vi "BlueSimpleReachTask 2.vi"() -> ()   [LabVIEW 2010]
uses:
  <vilib>/sound2/lvsound2.llb/Sound Data Format.ctl
  <vilib>/sound2/lvsound2.llb/Sampling Mode.ctl
  Controls/Bits to Write.ctl
  <vilib>/sound2/lvsound2.llb/Sound Output Set Volume (Single).vi
  <vilib>/sound2/lvsound2.llb/Sound Output Write (DBL Single).vi
  <vilib>/measure/NI_MABase.lvlib
panel:
  in  "Time to wait\nbefore treat \nArm freeze (S)":dbl=5.0
  in  "Arm Freeze \nCounter":bool
  in  "Volume":dbl(slide)=70.40816326530613 scale=0.0..100.0
  in  "Frequency":dbl=500.0 format="%0.2p"
  in  "error in (no error)":errorcluster
  in  "Sound Format":T1={"sample rate (S/s)"=44100.0, "number of channels"=2, "bits per sample"=16}
  in  "Number of Samples/ch":i32=5000
  in  "Device ID":u32
  in  "Catch Trial":bool
  in  "Catch probability":i32 min=0 max=100 step=1
  out "Catch Trial?":bool
  out "DO Task":refnum<k21>="BlueSimple_DO_All"
  out "DI Task":refnum<k21>="BlueSimple_DI"
  out "Exp correct":i32
  out "Record flag":bool
  in  "Recenter motor":bool
  in  "Override bumps":bool
  in  "Start bump timer?":bool
  in  "Trial type":u16(ring) items=["Allflash/sensory", "Precue/memory"]
  in  "DBS On?":bool
  in  "Home+target OK?":bool
  out "Exp reset":bool
  out "target set #":i32
  in  "duration (s)":dbl=0.18 format="%.4f"
  in  "Inter-pulse delay":cluster{"Fix":dbl, "Rnd":dbl}={"Fix"=0.0, "Rnd"=1.5} {"Rnd" format="%.4f"; "Fix" format="%_4g"}
  in  "Autofeed?":bool
  out "Just initialized\nhold loop?":bool
  in  "Home reward?":bool
  in  "Home  reward":cluster{"Fix":dbl, "Rnd":dbl} {"Rnd" format="%.4f"; "Fix" format="%_4g"}
  in  "Override 4":bool caption="Override 1"
  in  "Override 3":bool caption="Override 1"
  in  "Override 2":bool=TRUE caption="Override 1"
  in  "Override 1":bool=TRUE
  in  "LED lines":T2={"LED1"=1, "LED2"=2, "LED3"=3, "LED4"=4}
  in  "LED1":i16=5
  in  "LED2":i16=6
  in  "LED3":i16=7
  in  "LED4":i16=8
  in  "Bump Parameters":T3={"Distance (deg)"=2.0, "Travel time (ms)"=500.0} {"Travel time (ms)" min=0.1 max=10000.0; "Distance (deg)" min=0.1}
  in  "Bump delay":cluster{"Fix":dbl, "Rnd":dbl}={"Fix"=2.0, "Rnd"=8.0} {"Rnd" format="%.4f"; "Fix" format="%_4g"}
  in  "Sine parameters":T4={"Frequency"=1.0, "Degrees\npk-pk"=8.0, "Cycles"=10000} {"Degrees\npk-pk" min=0.1 max=120.0; "Frequency" min=0.001 format="%#_4g"}
  in  "Home":bool
  in  "Bumps":bool
  in  "Sines?":bool
  out "target set size":i32
  out "# target sets":u16
  in  "# Cycles":i16=20
  out "Instruct duration":dbl format="%.4f"
  out "Pre-I hold":dbl format="%.4f"
  out "Touching target\nlast time?":bool
  in  "Rand/Seq?":bool=TRUE
  in  "Target set":i16[](array[ring]) items=["1", "2", "3", "4"]
  in  "Block":T5(array[cluster])=array[6501 elements]
  in  "Settings In":T6={"Pre-I hold"={"Fixed (s)"=0.5, "Random (s)"=0.5}, "LED I duration"={"Fixed (s)"=0.5, "Random (s)"=0.0}, "All Flash?"=FALSE, "Pre-cue brightness"=0, "Post-I hold"={"Fixed (s)"=0.7, "Random (s)"=0.3}, "Post-I \nbounce-off"={"Fixed (s)"=0.3, "Random (s)"=0.0}, "Capture timeout"={"Fixed (s)"=1.5, "Random (s)"=0.0}, "Tone duration"={"Fixed (s)"=0.5, "Random (s)"=0.0}, "LED C duration"={"Fixed (s)"=0.5, "Random (s)"=0.0}, "Cue brightness"=0, "Hold duration"={"Fixed (s)"=0.3, "Random (s)"=0.0}, "Allowed\nbounce-off"={"Fixed (s)"=0.2, "Random (s)"=0.0}, "Post-capture brightness"=0, "Reward duration"={"Fixed (s)"=0.7, "Random (s)"=0.0}, "Intertrial interval"={"Fixed (s)"=0.5, "Random (s)"=0.0}, "Persistent Mode?"=FALSE, "Error bong?"=TRUE, "Critter"=0, "Blocks"=[], "Target set"=[], "Rand/Seq?"=TRUE, "Trial type"=0, "Sines?"=FALSE, "Bumps"=FALSE, "Sine parameters"={"Frequency"=0.25, "Degrees\npk-pk"=6.0, "Cycles"=10000}, "Bump timing"={"Fix"=2.0, "Rnd"=8.0}, "Bump Parameters"={"Distance (deg)"=2.0, "Travel time (ms)"=500.0}, "DBS On?"=FALSE, "Home reward?"=FALSE, "Home+target OK?"=FALSE} {"Bump Parameters"."Travel time (ms)" min=0.1 max=10000.0; "Bump Parameters"."Distance (deg)" min=0.1; "Bump timing"."Rnd" format="%.4f"; "Bump timing"."Fix" format="%_4g"; "Sine parameters"."Degrees\npk-pk" min=0.1 max=120.0; "Sine parameters"."Frequency" min=0.001 format="%#_4g"; "Trial type" items=["Allflash/sensory", "Precue/memory"]; "Target set" items=["1", "2", "3", "4"]; "Critter" items=["Mojo", "Smokey"]; "Post-I \nbounce-off"."Random (s)" format="%.4f"; "Post-I \nbounce-off"."Fixed (s)" format="%_4g"; "Allowed\nbounce-off"."Random (s)" format="%.4f"; "Allowed\nbounce-off"."Fixed (s)" format="%_4g"; "LED C duration"."Random (s)" format="%.4f"; "LED C duration"."Fixed (s)" format="%.4f"; "Capture timeout"."Random (s)" format="%.4f"; "Capture timeout"."Fixed (s)" format="%.4f"; "Post-I hold"."Random (s)" format="%.4f"; "Post-I hold"."Fixed (s)" format="%.4f"; "Hold duration"."Random (s)" format="%.4f"; "Hold duration"."Fixed (s)" format="%_4g"; "Intertrial interval"."Random (s)" format="%.4f"; "Intertrial interval"."Fixed (s)" format="%.4f"; "Reward duration"."Random (s)" format="%.4f"; "Reward duration"."Fixed (s)" format="%.4f"; "LED I duration"."Random (s)" format="%.4f"; "LED I duration"."Fixed (s)" format="%.4f"; "Tone duration"."Random (s)" format="%.4f"; "Tone duration"."Fixed (s)" format="%.4f"; "Pre-I hold"."Random (s)" format="%.4f"; "Pre-I hold"."Fixed (s)" format="%_4g"}
  in  "pause":bool
  out "Assign settings":bool
  out "current path":path
  out "next trial path":path
  in  "Critter":u16(ring) items=["Mojo", "Smokey", "Blue", "Odo", "Monk 5", "Monk 6", "Monk 7", "Monk 8", "Monk 9", "Monk 10"]
  out "Total incorrect":i32
  in  "Write Settings":bool
  in  "Read Settings":bool
  in  "All Flash?":bool
  in  "Post-capture brightness":i16 caption="Brightness"
  in  "Cue brightness":i16=6 caption="Brightness"
  in  "Pre-cue brightness":i16 caption="Brightness"
  out "Total correct":i32
  out "Total %":dbl
  out "Total trials":i32
  in  "Error\nbong?":bool=TRUE
  out "TS Home":bool
  out "TS 4":bool
  out "TS 3":bool
  out "TS 2":bool
  out "TS 1":bool
  out "Waveform Chart":T7(graph)
  out "Block trials":i32
  out "Block %":dbl
  in  "Reset\ncounters":bool
  in  "Post-I \nbounce-off":cluster{"Fix":dbl, "Rnd":dbl}={"Fix"=0.3, "Rnd"=0.0} caption="Allowed\nbounce-off" {"Rnd" format="%.4f"; "Fix" format="%_4g"}
  out "Exp trials":i32
  out "Exp %":dbl
  in  "Touch lines":T8={"Home touch"=0, "Touch 1"=1, "Touch 2"=2, "Touch 3"=3, "Touch 4"=4}
  out "Current stage":T9(ring)
  in  "Allowed\nbounce-off":cluster{"Fix":dbl, "Rnd":dbl}={"Fix"=0.2, "Rnd"=0.0} {"Rnd" format="%.4f"; "Fix" format="%_4g"}
  in  "LED C duration":cluster{"Fix":dbl, "Rnd":dbl}={"Fix"=0.5, "Rnd"=0.0} caption="LED duration" {"Rnd" format="%.4f"; "Fix" format="%.4f"}
  in  "Capture timeout":cluster{"Fix":dbl, "Rnd":dbl}={"Fix"=1.5, "Rnd"=0.0} caption="Response time" {"Rnd" format="%.4f"; "Fix" format="%.4f"}
  in  "Post-I hold":cluster{"Fix":dbl, "Rnd":dbl}={"Fix"=0.5, "Rnd"=0.5} {"Rnd" format="%.4f"; "Fix" format="%.4f"}
  out "Last trial successful?":bool
  in  "Persistent\n Mode?":bool
  in  "Touch 4":i16=4
  in  "Touch 3":i16=3
  in  "Touch 2":i16=2
  in  "Touch 1":i16=1
  in  "Home touch":i16
  in  "Hold duration":cluster{"Fix":dbl, "Rnd":dbl}={"Fix"=0.3, "Rnd"=0.0} {"Rnd" format="%.4f"; "Fix" format="%_4g"}
  out "Target":i16
  in  "stop":bool
  in  "device":i16=1
  in  "line direction map":i32=2147483616 format="%.0b"
  out "DIGIO task ID":u32 format="%.0x"
  out "error out":errorcluster
  in  "Intertrial interval":cluster{"Fix":dbl, "Rnd":dbl}={"Fix"=0.5, "Rnd"=0.0} {"Rnd" format="%.4f"; "Fix" format="%.4f"}
  in  "Reward duration":cluster{"Fix":dbl, "Rnd":dbl}={"Fix"=0.7, "Rnd"=0.0} {"Rnd" format="%.4f"; "Fix" format="%.4f"}
  in  "LED I duration":cluster{"Fix":dbl, "Rnd":dbl}={"Fix"=0.5, "Rnd"=0.0} caption="LED duration" {"Rnd" format="%.4f"; "Fix" format="%.4f"}
  in  "Tone duration":cluster{"Fix":dbl, "Rnd":dbl}={"Fix"=0.5, "Rnd"=0.0} {"Rnd" format="%.4f"; "Fix" format="%.4f"}
  in  "Pre-I hold":cluster{"Fix":dbl, "Rnd":dbl}={"Fix"=0.5, "Rnd"=0.5} {"Rnd" format="%.4f"; "Fix" format="%_4g"}
  # "Auto-feed"
  # "DBS"
  # "Pre-\ninstruction\nhold"
  # "Post-\ninstruction\nhold"
  # "Instruction"
  # "Target capture"
  # "Target hold"
  # "Reward"
  # "Intertrial"
  # "Motor"
  # "Override"
  # "Home key tone"
  # "+"
  # "+"
  # "+"
  # "Pre-\ninstruction\nhold"
  # "Instruction"
  # "Post-\ninstruction\nhold"
  # "Target capture"
  # "Target hold"
  # "Reward"
  # "Intertrial"
  # "+"
  # "+"
  # "+"
  # "+"
  # "+"
  # "+"
  # "+"
  # "+"
  # "+"
  # "+"
  # "+"
  # "+"
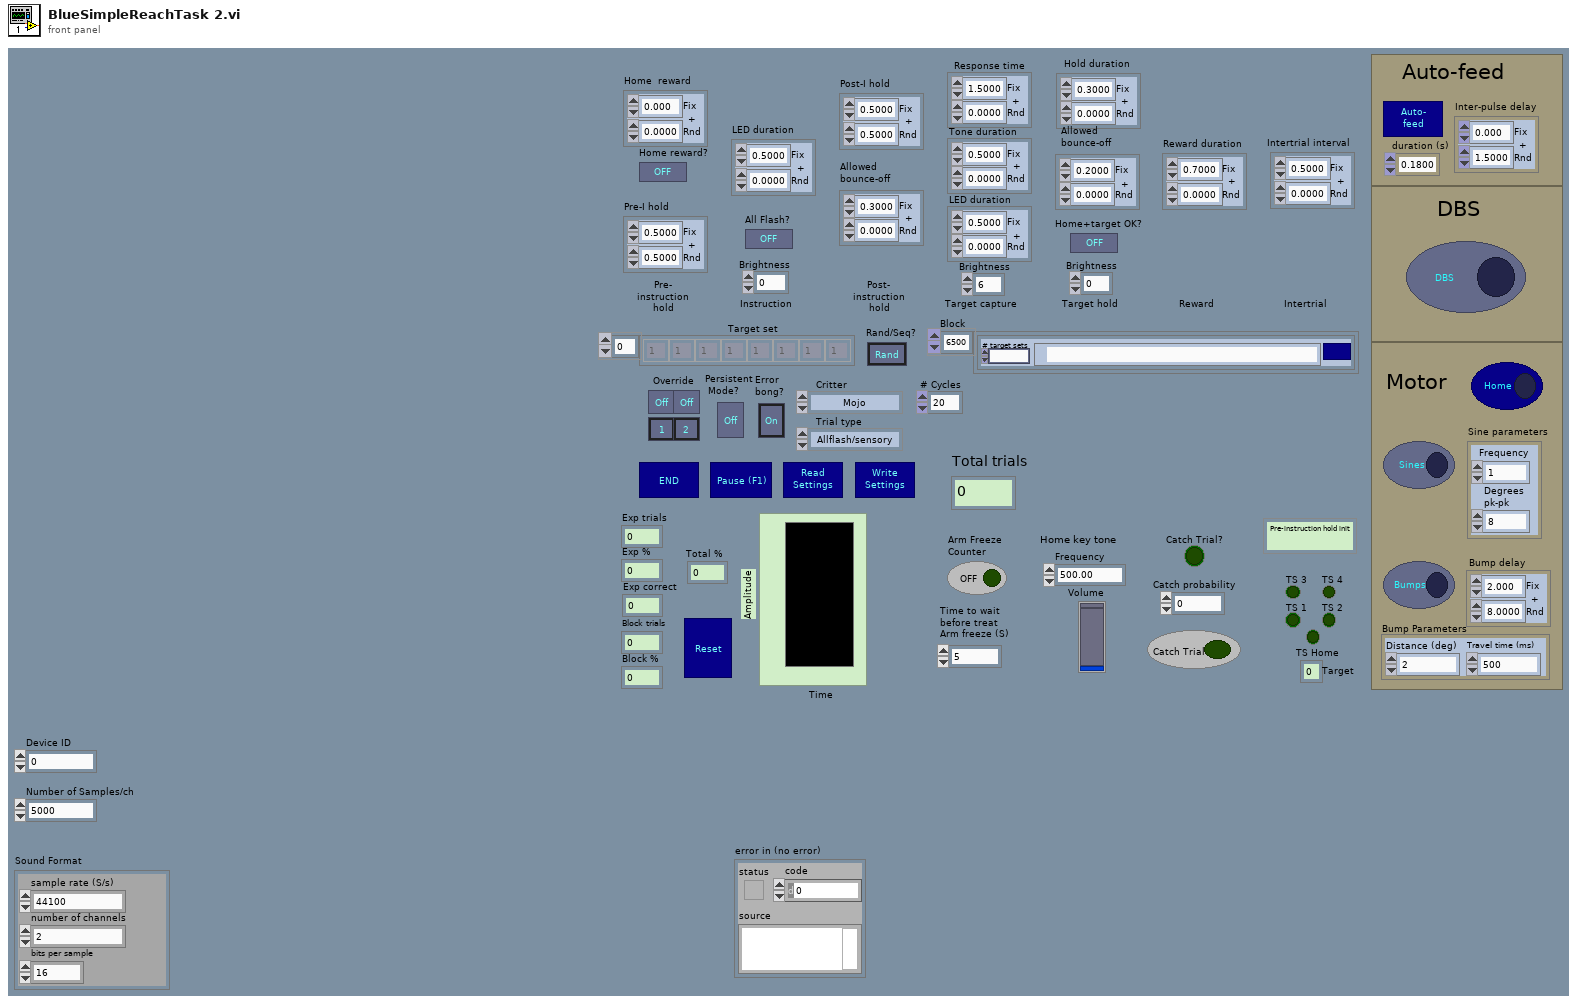
[diagram p1: front panel]
types:
  T1 = typedef "Sound Data Format.ctl" = cluster{"sample rate (S/s)":dbl, "number of channels":i32, "bits per sample":i32}
  T2 = cluster{"LED1":i16, "LED2":i16, "LED3":i16, "LED4":i16}
  T3 = cluster{"Distance (deg)":dbl, "Travel time (ms)":dbl}
  T4 = cluster{"Frequency":dbl, "Degrees\npk-pk":dbl, "Cycles":i16}
  T5 = cluster{"Settings file":path, "# target sets":u16}[]
  T6 = cluster{"Pre-I hold":cluster{"Fixed (s)":dbl, "Random (s)":dbl}, "LED I duration":cluster{"Fixed (s)":dbl, "Random (s)":dbl}, "All Flash?":bool, "Pre-cue brightness":i16, "Post-I hold":cluster{"Fixed (s)":dbl, "Random (s)":dbl}, "Post-I \nbounce-off":cluster{"Fixed (s)":dbl, "Random (s)":dbl}, "Capture timeout":cluster{"Fixed (s)":dbl, "Random (s)":dbl}, "Tone duration":cluster{"Fixed (s)":dbl, "Random (s)":dbl}, "LED C duration":cluster{"Fixed (s)":dbl, "Random (s)":dbl}, "Cue brightness":i16, "Hold duration":cluster{"Fixed (s)":dbl, "Random (s)":dbl}, "Allowed\nbounce-off":cluster{"Fixed (s)":dbl, "Random (s)":dbl}, "Post-capture brightness":i16, "Reward duration":cluster{"Fixed (s)":dbl, "Random (s)":dbl}, "Intertrial interval":cluster{"Fixed (s)":dbl, "Random (s)":dbl}, "Persistent Mode?":bool, "Error bong?":bool, "Critter":u16, "Blocks":cluster{"Settings file":path, "# target sets":dbl}[], "Target set":i16[], "Rand/Seq?":bool, "Trial type":u16, "Sines?":bool, "Bumps":bool, "Sine parameters":cluster{"Frequency":dbl, "Degrees\npk-pk":dbl, "Cycles":i16}, "Bump timing":cluster{"Fix":dbl, "Rnd":dbl}, "Bump Parameters":cluster{"Distance (deg)":dbl, "Travel time (ms)":dbl}, "DBS On?":bool, "Home reward?":bool, "Home+target OK?":bool}
  T7 = cluster{"Segment Percentage":dbl, "Total % correct":dbl}
  T8 = cluster{"Home touch":i16, "Touch 1":i16, "Touch 2":i16, "Touch 3":i16, "Touch 4":i16}
  T9 = enum16{"Pre-instruction hold init", "Pre-instruction hold", "Instruction init", "Instruction", "Post-instruction hold init", "Post-instruction hold", "Target capture init", "Target capture", "Target hold init", "Target hold", "Reward stage", "Intertrial"}
  T10 = typedef "Sampling Mode.ctl" = i32
  T11 = typedef "Sound Output Task ID.ctl" = u32
  T12 = typedef "Bits to Write.ctl" = enum16{"LED 1 on", "LED 1 off", "LED 2 on", "LED 2 off", "LED 3 on", "LED 3 off", "LED 4 on", "LED 4 off", "All LEDs on", "All LEDs off", "In trial on", "In trial off", "Buzzer on", "Buzzer off", "Reward on", "Reward off", "Target number", "Trial type preQ on", "Trial type preQ off", "Error on", "Error off", "Trial number", "DBS on", "DBS off", "Sine on", "Sine off", "All Bits On", "All Bits Off", "Init", "Specify mask/pattern"}
  T13 = enum16{"Reset", "Increment", "Reset for exp", "Initialize"}
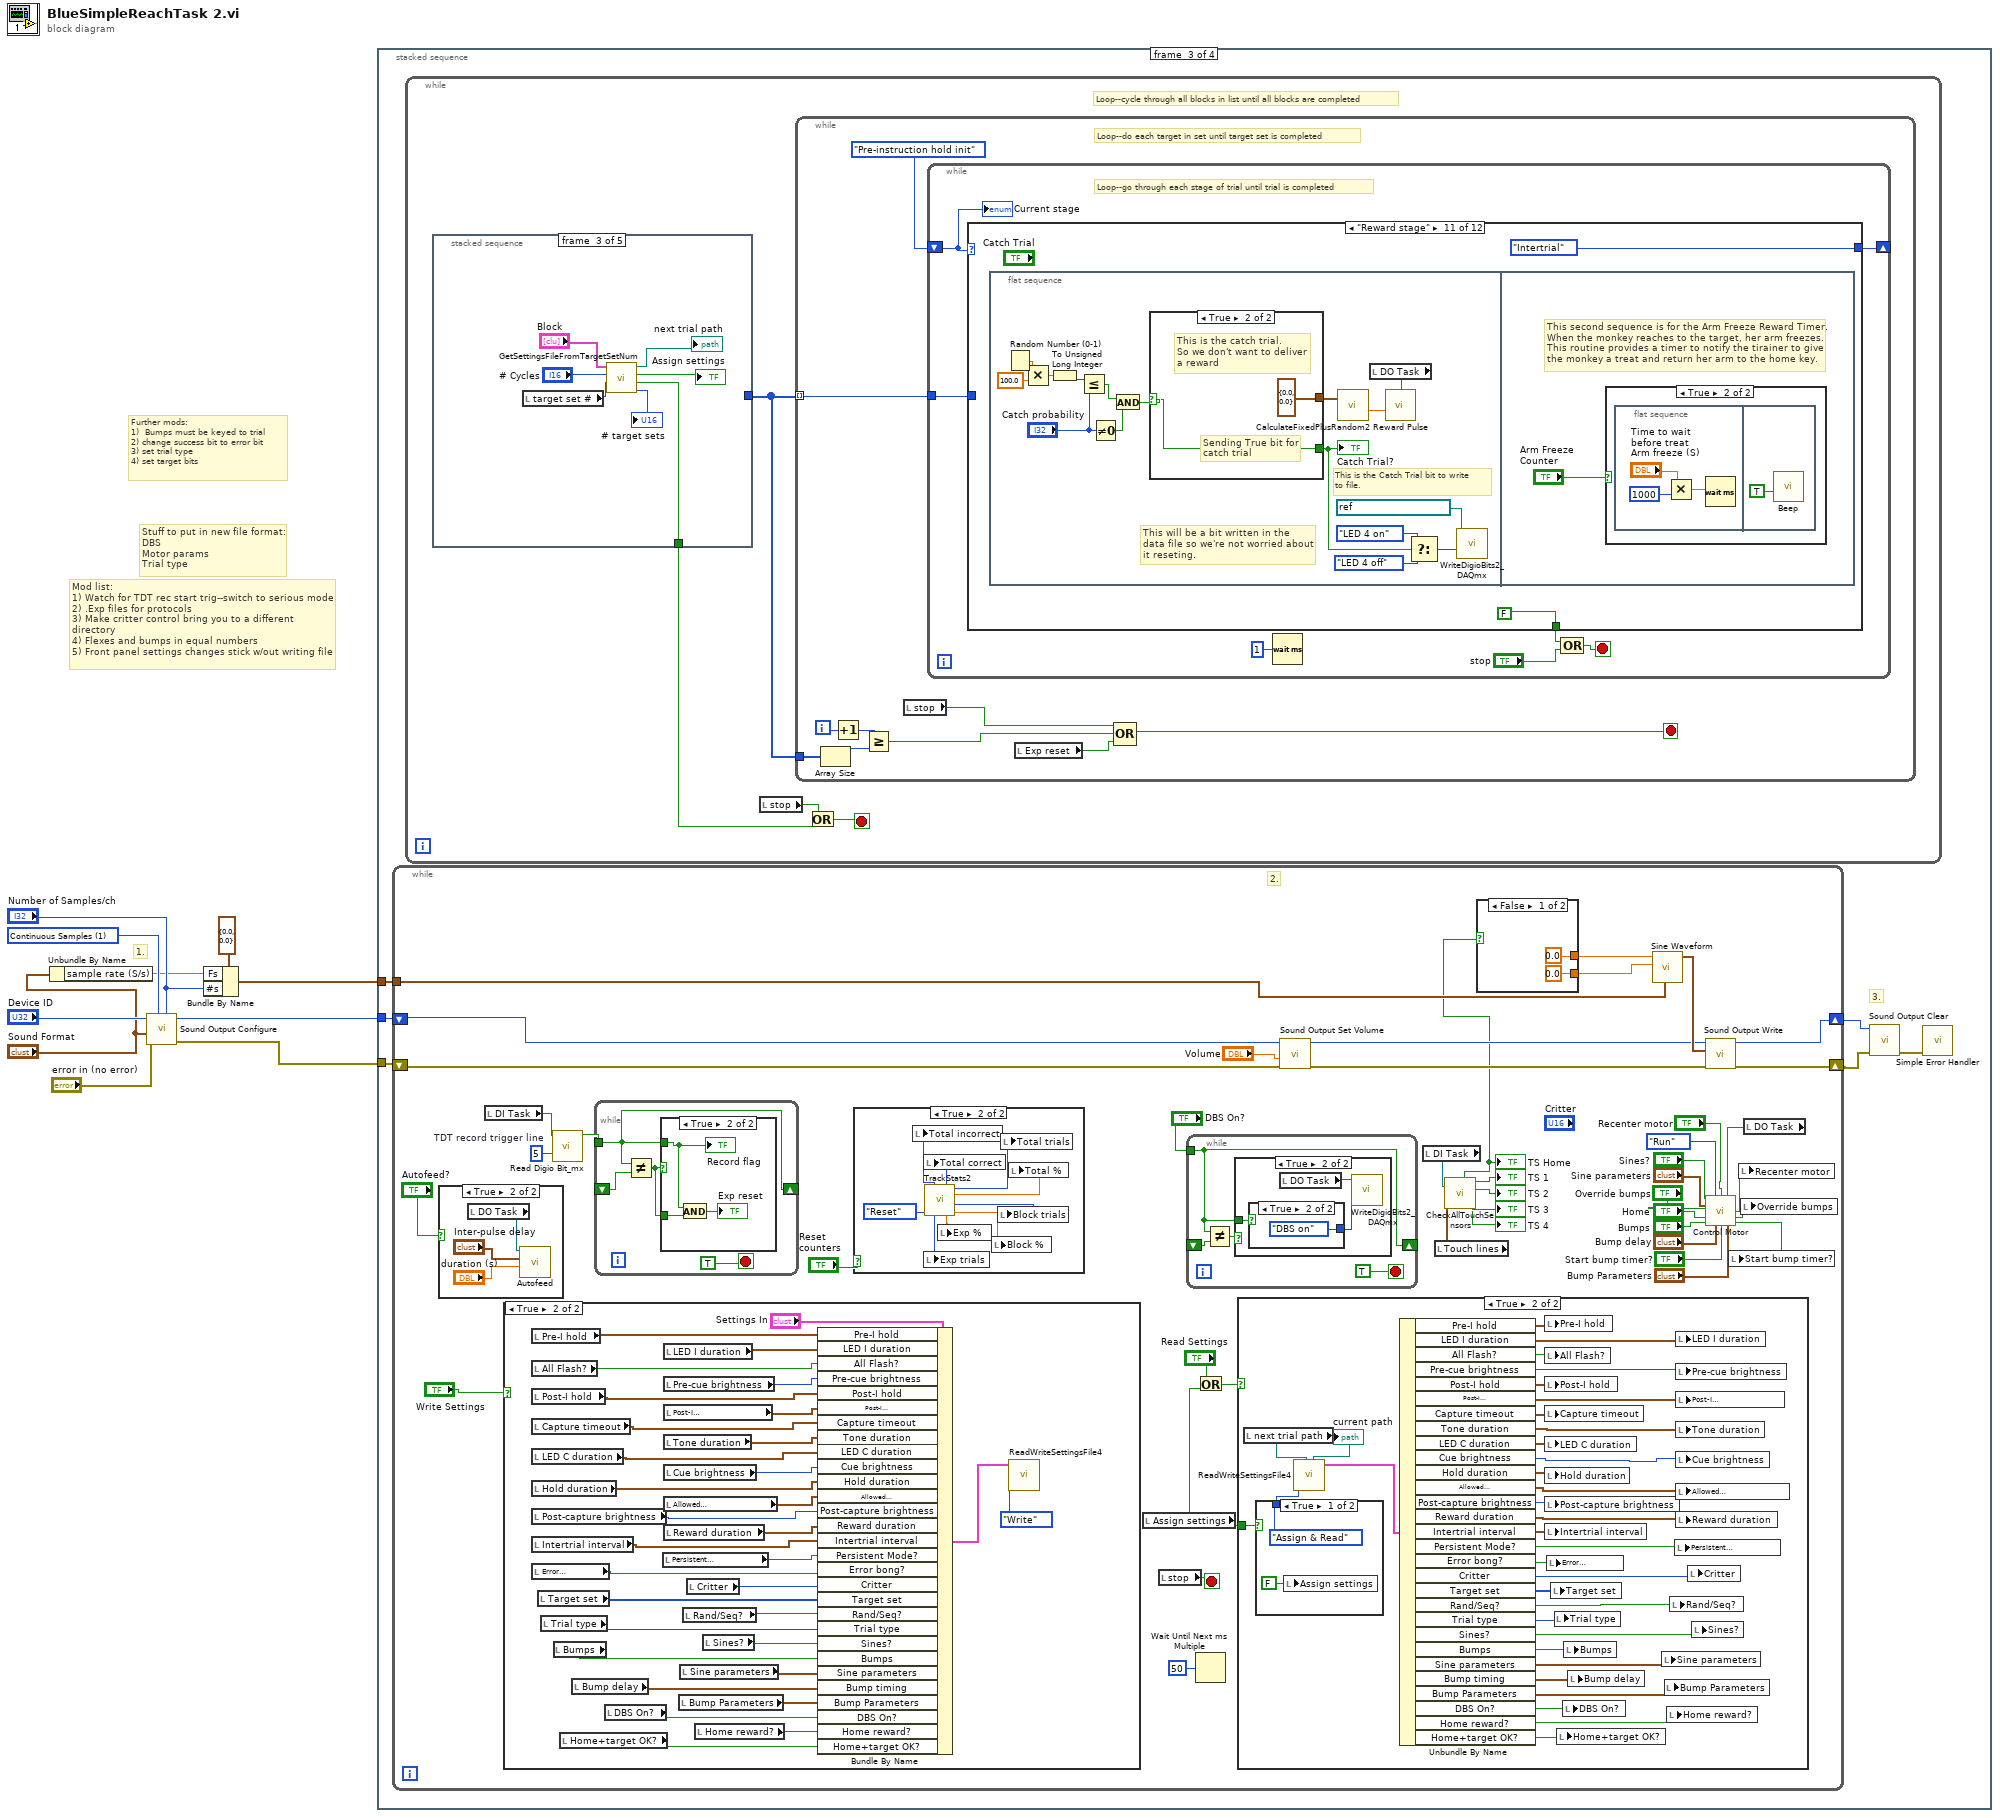
[diagram p0: block diagram]
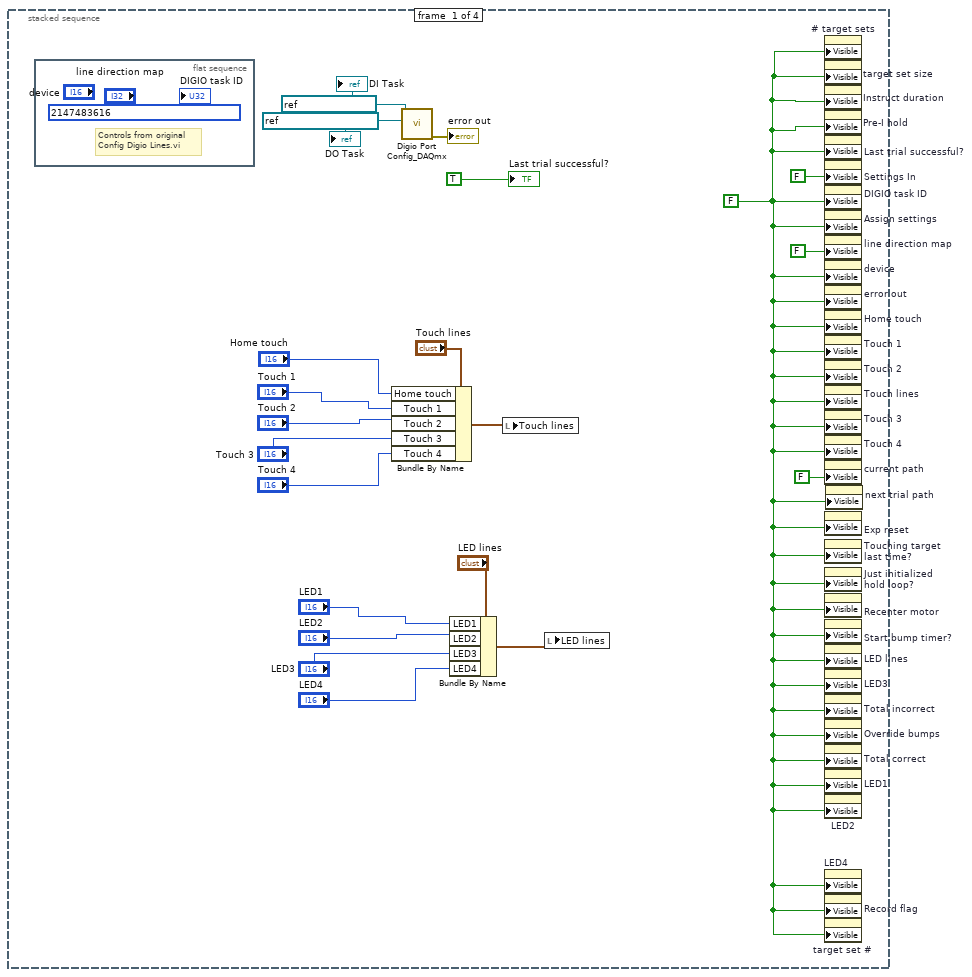
[diagram p2: hidden frame]
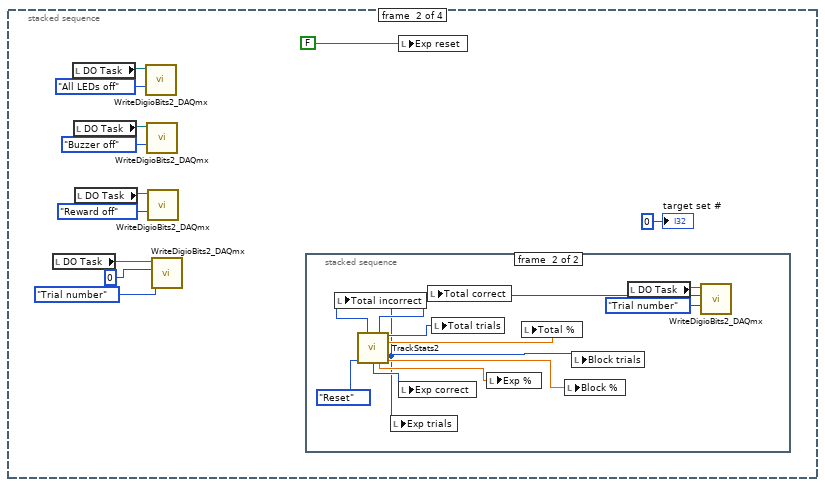
[diagram p3: hidden frame]
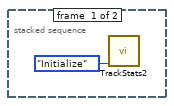
[diagram p4: hidden frame]
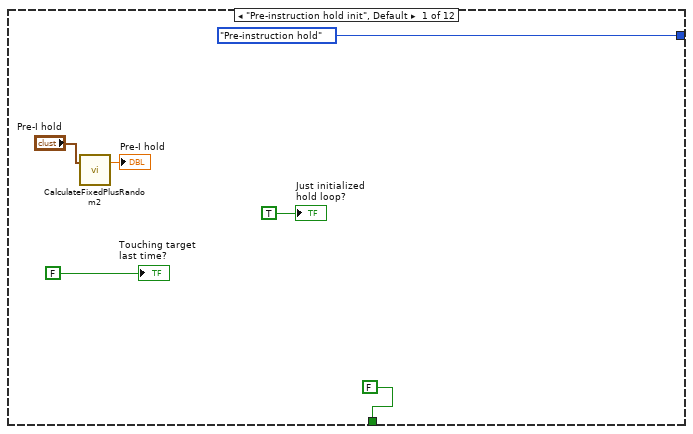
[diagram p5: hidden frame]
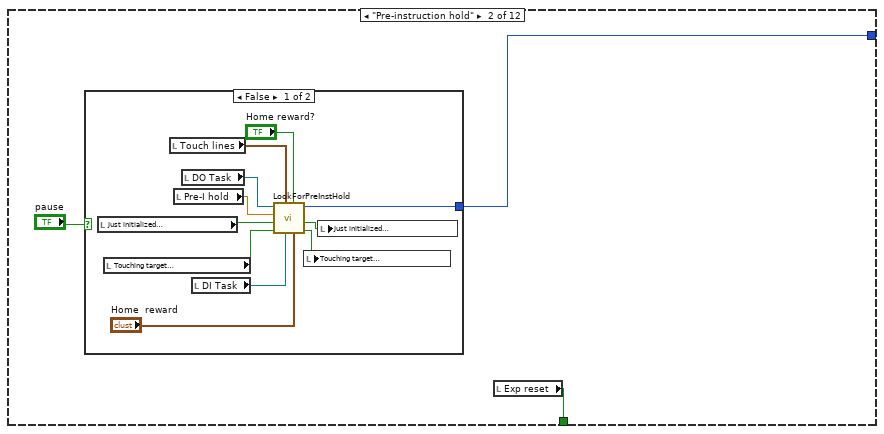
[diagram p6: hidden frame]
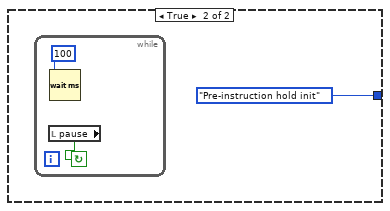
[diagram p7: hidden frame]
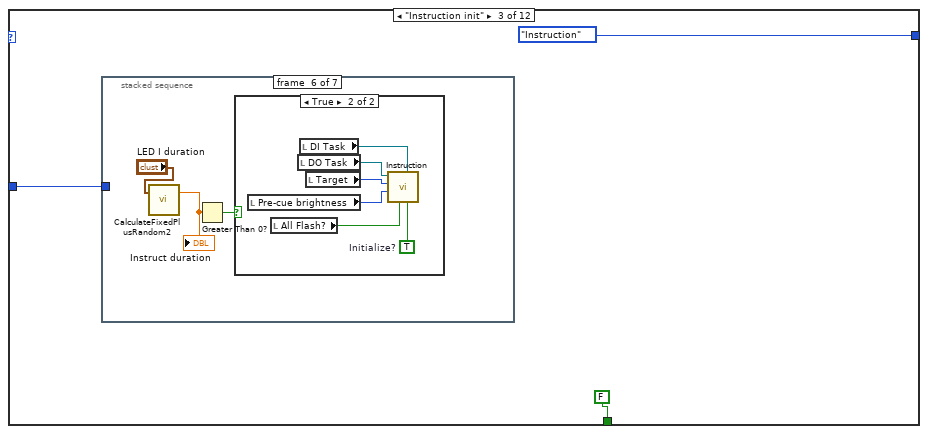
[diagram p8: hidden frame]
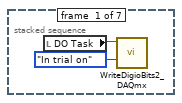
[diagram p9: hidden frame]
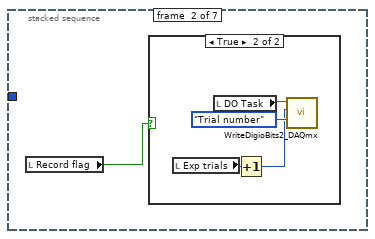
[diagram p10: hidden frame]
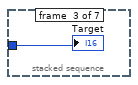
[diagram p12: hidden frame]
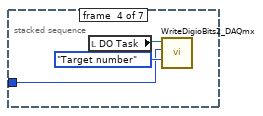
[diagram p13: hidden frame]
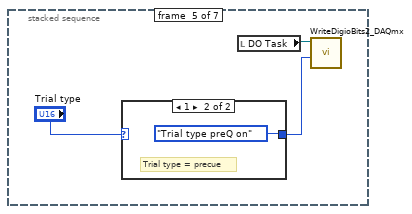
[diagram p14: hidden frame]
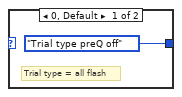
[diagram p15: hidden frame]
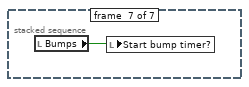
[diagram p17: hidden frame]
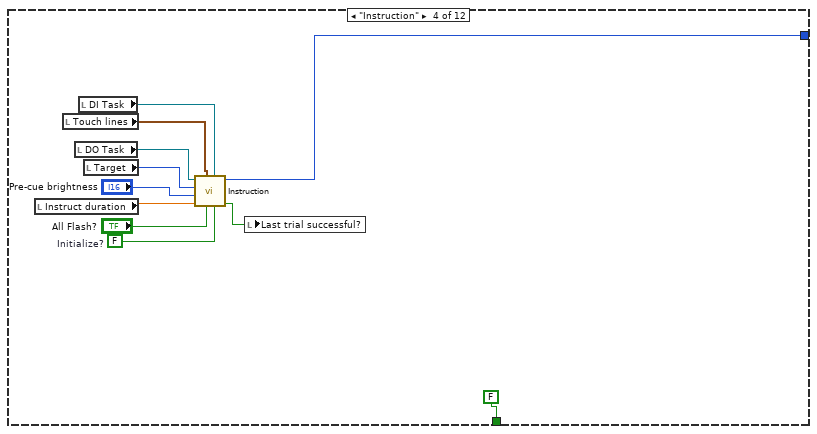
[diagram p18: hidden frame]
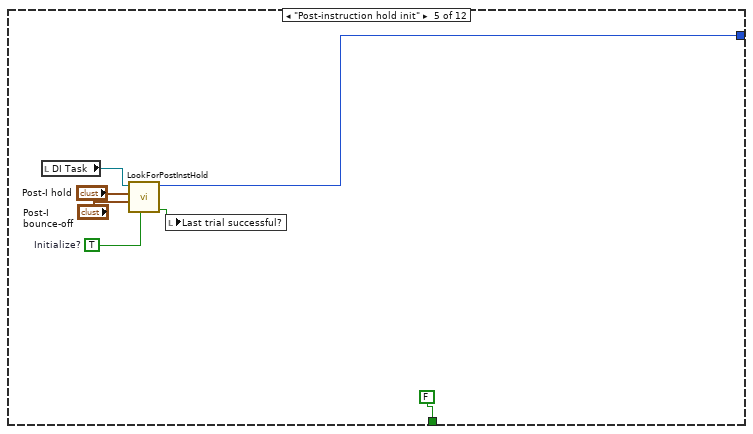
[diagram p19: hidden frame]
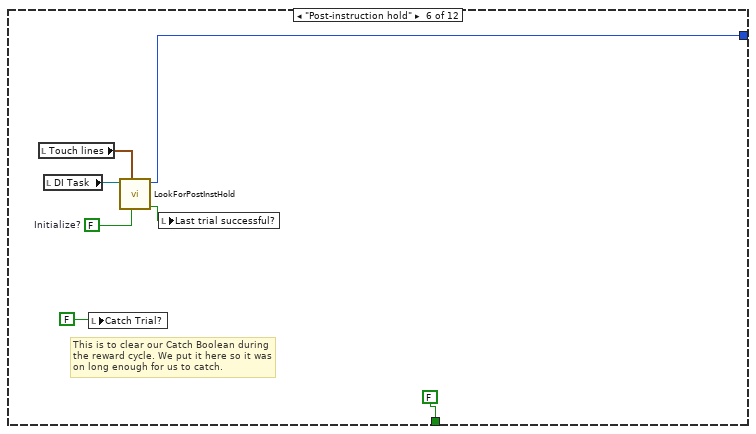
[diagram p20: hidden frame]
diagram:
  w9 = T10 1 items=["Finite Samples", "Continuous Samples"] ("sample mode")
  # "1."
  # "Stuff to put in new file format:\nDBS\nMotor params\nTrial type"
  # "Further mods:\n1)  Bumps must be keyed to trial\n2) change success bit to error bit\n3) set trial type\n4) set target bits"
  # "Mod list:\n1) Watch for TDT rec start trig--switch to serious mode\n2) .Exp files for protocols\n3) Make critter control bring you to a different directory\n4) Flexes and bumps in equal numbers\n5) Front panel settings changes stick w/out writing file"
  n1 = Unbundle By Name("Sound Format") -> ("sample rate (S/s)"=w6:dbl)
  n2 = call <vilib>:"Sound Output Configure.vi"("number of samples/ch"="Number of Samples/ch", "sample mode"=w9, "error in (no error)"="error in (no error)", "sound format"="Sound Format", "device ID"="Device ID") -> ("error out"=w3:errorcluster, "task ID"=w2:T11)  [unwired: 5 in]
  n3 = Bundle By Name(cluster=cluster{"Fs":dbl, "#s":dbl} {"Fs"=0.0, "#s"=0.0} ("sampling info"), "Fs"=w6, "#s"="Number of Samples/ch") -> (w1:cluster{"Fs":dbl, "#s":dbl})
  n4 = stacked-sequence {
    tunnel: w3 -> [_ _ w61 _]
    tunnel: w2 -> [_ _ w60 _]
    tunnel: w1 -> [_ _ w59 _]
    frame #0 {
      w12 = refnum<k21> "BlueSimple_DO_All" ("DO Task")
      w13 = refnum<k21> "BlueSimple_DI" ("DI Task")
      w14 = FALSE ("Persistent Mode?")
      n5 = flat-sequence {
        frame #0 {
          (unwired) 2147483616 ("line direction map")
          # "Controls from original\nConfig Digio Lines.vi"
        }
      }
      n6 = Bundle By Name(cluster="Touch lines", "Home touch"="Home touch", "Touch 1"="Touch 1", "Touch 2"="Touch 2", "Touch 3"="Touch 3", "Touch 4"="Touch 4") -> (w30:T8)
      n7 = call "Digio Port Config_DAQmx.vi"("DO Task"=w12, "DI Task"=w13) -> ("error out"=→"error out":errorcluster)  [unwired: 7 in]
      n8 = Bundle By Name(cluster="LED lines", "LED1"="LED1", "LED2"="LED2", "LED3"="LED3", "LED4"="LED4") -> (w18:T2)
      n9 = local write "Touch lines"(w30) -> ()
      n10 = local write "LED lines"(w18) -> ()
      n11 = property on="# target sets" class="DigNum (strict)"("Visible"=w14) -> ()  [unwired: 2 in, 2 out]
      n12 = property on="target set size" class="DigNum (strict)"("Visible"=w14) -> ()  [unwired: 2 in, 2 out]
      n13 = property on="Instruct duration" class="DigNum (strict)"("Visible"=w14) -> ()  [unwired: 2 in, 2 out]
      n14 = property on="Pre-I hold" class="DigNum (strict)"("Visible"=w14) -> ()  [unwired: 2 in, 2 out]
      n15 = property on="Last trial successful?" class="Bool (strict)"("Visible"=w14) -> ()  [unwired: 2 in, 2 out]
      n16 = property on="Settings In" class="Clust (strict)"("Visible"=FALSE) -> ()  [unwired: 2 in, 2 out]
      n17 = property on="DIGIO task ID" class="DigNum (strict)"("Visible"=w14) -> ()  [unwired: 2 in, 2 out]
      n18 = property on="Assign settings" class="Bool (strict)"("Visible"=w14) -> ()  [unwired: 2 in, 2 out]
      n19 = property on="line direction map" class="DigNum (strict)"("Visible"=FALSE) -> ()  [unwired: 2 in, 2 out]
      n20 = property on="device" class="DigNum (strict)"("Visible"=w14) -> ()  [unwired: 2 in, 2 out]
      n21 = property on="error out" class="Clust (strict)"("Visible"=w14) -> ()  [unwired: 2 in, 2 out]
      n22 = property on="Home touch" class="DigNum (strict)"("Visible"=w14) -> ()  [unwired: 2 in, 2 out]
      n23 = property on="Touch 1" class="DigNum (strict)"("Visible"=w14) -> ()  [unwired: 2 in, 2 out]
      n24 = property on="Touch 2" class="DigNum (strict)"("Visible"=w14) -> ()  [unwired: 2 in, 2 out]
      n25 = property on="Touch lines" class="Clust (strict)"("Visible"=w14) -> ()  [unwired: 2 in, 2 out]
      n26 = property on="Touch 3" class="DigNum (strict)"("Visible"=w14) -> ()  [unwired: 2 in, 2 out]
      n27 = property on="Touch 4" class="DigNum (strict)"("Visible"=w14) -> ()  [unwired: 2 in, 2 out]
      n28 = property on="current path" class="Path"("Visible"=FALSE) -> ()  [unwired: 2 in, 2 out]
      n29 = property on="Exp reset" class="Bool (strict)"("Visible"=w14) -> ()  [unwired: 2 in, 2 out]
      n30 = property on="Touching target\nlast time?" class="Bool (strict)"("Visible"=w14) -> ()  [unwired: 2 in, 2 out]
      n31 = property on="Just initialized\nhold loop?" class="Bool (strict)"("Visible"=w14) -> ()  [unwired: 2 in, 2 out]
      n32 = property on="Recenter motor" class="Bool (strict)"("Visible"=w14) -> ()  [unwired: 2 in, 2 out]
      n33 = property on="Start bump timer?" class="Bool (strict)"("Visible"=w14) -> ()  [unwired: 2 in, 2 out]
      n34 = property on="LED lines" class="Clust (strict)"("Visible"=w14) -> ()  [unwired: 2 in, 2 out]
      n35 = property on="LED3" class="DigNum (strict)"("Visible"=w14) -> ()  [unwired: 2 in, 2 out]
      n36 = property on="Total incorrect" class="DigNum (strict)"("Visible"=w14) -> ()  [unwired: 2 in, 2 out]
      n37 = property on="Override bumps" class="Bool (strict)"("Visible"=w14) -> ()  [unwired: 2 in, 2 out]
      n38 = property on="Total correct" class="DigNum (strict)"("Visible"=w14) -> ()  [unwired: 2 in, 2 out]
      n39 = property on="LED1" class="DigNum (strict)"("Visible"=w14) -> ()  [unwired: 2 in, 2 out]
      n40 = property on="LED2" class="DigNum (strict)"("Visible"=w14) -> ()  [unwired: 2 in, 2 out]
      n41 = property on="LED4" class="DigNum (strict)"("Visible"=w14) -> ()  [unwired: 2 in, 2 out]
      n42 = property on="Record flag" class="Bool (strict)"("Visible"=w14) -> ()  [unwired: 2 in, 2 out]
      n43 = property on="target set #" class="DigNum (strict)"("Visible"=w14) -> ()  [unwired: 2 in, 2 out]
      n44 = property on="next trial path" class="Path"("Visible"=w14) -> ()  [unwired: 2 in, 2 out]
      "Last trial successful?" <- TRUE ("Persistent Mode?")
      "DI Task" <- w13
      "DO Task" <- w12
    }
    frame #1 {
      n45 = local read "DO Task"() -> (w40:refnum<k21>)
      n46 = local read "DO Task"() -> (w33:refnum<k21>)
      n47 = local read "DO Task"() -> (w34:refnum<k21>)
      n48 = local read "DO Task"() -> (w36:refnum<k21>)
      n49 = call "WriteDigioBits2_DAQmx.vi"("Bits to write"=Bits_to_Write."All LEDs off", "DO Task"=w33) -> ()  [unwired: 9 in, 1 out]
      n50 = call "WriteDigioBits2_DAQmx.vi"("Bits to write"=Bits_to_Write."Buzzer off", "DO Task"=w34) -> ()  [unwired: 9 in, 1 out]
      n51 = call "WriteDigioBits2_DAQmx.vi"("Bits to write"=Bits_to_Write."Reward off", "DO Task"=w36) -> ()  [unwired: 9 in, 1 out]
      n52 = call "WriteDigioBits2_DAQmx.vi"("Bits to write"=Bits_to_Write."Trial number", "Number"=u32 0, "DO Task"=w40) -> ()  [unwired: 8 in, 1 out]
      n53 = stacked-sequence {
        frame #0 {
          n54 = call "TrackStats2.vi"("Command"=T13."Initialize") -> ()  [unwired: 6 in, 9 out]
        }
        frame #1 {
          n55 = call "TrackStats2.vi"("Command"=T13."Reset") -> ("Total incorrect"=w55:i32, "Total correct"=w54:i32, "# total trials"=w53:i32, "Total % correct"=w52:dbl, "Segment trials"=w48:i32, "Experiment trials"=w44:i32, "Experiment correct"=w47:i32, "Experiment %"=w50:dbl, "Segment Percentage"=w51:dbl)  [unwired: 6 in]
          n56 = local write "Total incorrect"(w55) -> ()
          n57 = local write "Exp trials"(w44) -> ()
          n58 = local write "Exp correct"(w47) -> ()
          n59 = local write "Total correct"(w54) -> ()
          n60 = local write "Total trials"(w53) -> ()
          n61 = local write "Exp %"(w50) -> ()
          n62 = local write "Total %"(w52) -> ()
          n63 = local write "Block %"(w51) -> ()
          n64 = local write "Block trials"(w48) -> ()
          n65 = local read "DO Task"() -> (w46:refnum<k21>)
          n66 = call "WriteDigioBits2_DAQmx.vi"("Bits to write"=Bits_to_Write."Trial number", "Number"=w44, "DO Task"=w46) -> ()  [unwired: 8 in, 1 out]
        }
      }
      n67 = local write "Exp reset"(FALSE ("Exp reset")) -> ()
      "target set #" <- 0 ("target set #")
    }
    frame #2 {
      # "3."
      n68 = while {
        shift-right: [w304] -> w57
        shift-left: w60 -> [w306]
        shift-right: [w303] -> w56
        shift-left: w61 -> [w305]
        tunnel: w59 -> [w307]
        stop <- w343 stop-if-true
        w315 = i16 5  # TDT record trigger line
        # "2."
        n69 = case shown="True" "Autofeed?" {
          frame False {
          }
          frame True {
            n70 = local read "DO Task"() -> (w357:refnum<k21>)
            n71 = call "Autofeed.vi"("duration"="duration (s)", "Auto-feed"="Inter-pulse delay", "DO Task"=w357) -> ()  [unwired: 4 in]
          }
        }
        n72 = local read "DI Task"() -> (w314:refnum<k21>)
        n73 = case shown="True" "Write Settings" {
          frame False {
          }
          frame True {
            n74 = local read "Pre-I hold"() -> (w398:cluster{"Fix":dbl, "Rnd":dbl})
            n75 = local read "All Flash?"() -> (w396:bool)
            n76 = local read "Post-I hold"() -> (w394:cluster{"Fix":dbl, "Rnd":dbl})
            n77 = local read "Capture timeout"() -> (w392:cluster{"Fix":dbl, "Rnd":dbl})
            n78 = local read "LED C duration"() -> (w390:cluster{"Fix":dbl, "Rnd":dbl})
            n79 = local read "Hold duration"() -> (w388:cluster{"Fix":dbl, "Rnd":dbl})
            n80 = local read "Post-capture brightness"() -> (w386:i16)
            n81 = local read "Intertrial interval"() -> (w384:cluster{"Fix":dbl, "Rnd":dbl})
            n82 = local read "Error\nbong?"() -> (w382:bool)
            n83 = local read "Target set"() -> (w378:i16[])
            n84 = local read "Trial type"() -> (w375:u16)
            n85 = local read "Bumps"() -> (w373:bool)
            n86 = local read "Home+target OK?"() -> (w367:bool)
            n87 = local read "Bump delay"() -> (w371:cluster{"Fix":dbl, "Rnd":dbl})
            n88 = local read "DBS On?"() -> (w369:bool)
            n89 = local read "Persistent\n Mode?"() -> (w383:bool)
            n90 = local read "LED I duration"() -> (w397:cluster{"Fix":dbl, "Rnd":dbl})
            n91 = local read "Pre-cue brightness"() -> (w395:i16)
            n92 = local read "Post-I \nbounce-off"() -> (w393:cluster{"Fix":dbl, "Rnd":dbl})
            n93 = local read "Tone duration"() -> (w391:cluster{"Fix":dbl, "Rnd":dbl})
            n94 = local read "Cue brightness"() -> (w389:i16)
            n95 = local read "Allowed\nbounce-off"() -> (w387:cluster{"Fix":dbl, "Rnd":dbl})
            n96 = local read "Reward duration"() -> (w385:cluster{"Fix":dbl, "Rnd":dbl})
            n97 = local read "Bump Parameters"() -> (w370:T3)
            n98 = local read "Sine parameters"() -> (w372:T4)
            n99 = local read "Rand/Seq?"() -> (w377:bool)
            n100 = local read "Critter"() -> (w379:u16)
            n101 = local read "Home reward?"() -> (w368:bool)
            n102 = local read "Sines?"() -> (w374:bool)
            n103 = Bundle By Name(cluster="Settings In", "Pre-I hold"=w398, "LED I duration"=w397, "All Flash?"=w396, "Pre-cue brightness"=w395, "Post-I hold"=w394, "Post-I \nbounce-off"=w393, "Capture timeout"=w392, "Tone duration"=w391, "LED C duration"=w390, "Cue brightness"=w389, "Hold duration"=w388, "Allowed\nbounce-off"=w387, "Post-capture brightness"=w386, "Reward duration"=w385, "Intertrial interval"=w384, "Persistent Mode?"=w383, "Error bong?"=w382, "Critter"=w379, "Target set"=w378, "Rand/Seq?"=w377, "Trial type"=w375, "Sines?"=w374, "Bumps"=w373, "Sine parameters"=w372, "Bump timing"=w371, "Bump Parameters"=w370, "DBS On?"=w369, "Home reward?"=w368, "Home+target OK?"=w367) -> (w376:T6)
            n104 = call "ReadWriteSettingsFile4.vi"("Read/write"=enum16{"Query & Read", "Assign & Read", "Write"}."Write", "Settings In"=w376) -> ()  [unwired: 4 in, 4 out]
          }
        }
        n105 = call "Read Digio Bit_mx.vi"("line"=w315, "DI Task"=w314) -> ("line state"=w313:bool)  [unwired: 7 in, 1 out]
        n106 = while {
          tunnel: w313 -> [w361]
          shift-right: [w361] -> _
          shift-left: _ -> [w362]
          stop <- TRUE stop-if-true
          n107 = Not Equal?(x=w361, y=w362) -> (x != y?=w360:bool)
          n108 = case shown="True" w360 {
            tunnel: w361 -> [_ w364]
            tunnel: w360 -> [_ w365]
            frame False {
            }
            frame True {
              n109 = And(x=w364, y=w365) -> (x .and. y?=→"Exp reset":bool)
              "Record flag" <- w364
            }
          }
        }
        n110 = case shown="True" "Reset\ncounters" {
          frame False {
          }
          frame True {
            n111 = call "TrackStats2.vi"("Command"=T13."Reset") -> ("Total incorrect"=w444:i32, "Total correct"=w443:i32, "# total trials"=w442:i32, "Total % correct"=w441:dbl, "Segment trials"=w440:i32, "Experiment trials"=w437:i32, "Experiment %"=w438:dbl, "Segment Percentage"=w439:dbl)  [unwired: 6 in, 1 out]
            n112 = local write "Total incorrect"(w444) -> ()
            n113 = local write "Total correct"(w443) -> ()
            n114 = local write "Exp trials"(w437) -> ()
            n115 = local write "Exp %"(w438) -> ()
            n116 = local write "Block %"(w439) -> ()
            n117 = local write "Block trials"(w440) -> ()
            n118 = local write "Total trials"(w442) -> ()
            n119 = local write "Total %"(w441) -> ()
          }
        }
        n120 = local read "Assign settings"() -> (w333:bool)
        n121 = local read "stop"() -> (w343:bool)
        n122 = while {
          shift-right: [w349] -> _
          shift-left: _ -> [w350]
          tunnel: "DBS On?" -> [w349]
          stop <- TRUE stop-if-true
          n123 = Not Equal?(x=w349, y=w350) -> (x != y?=w348:bool)
          n124 = case shown="True" w348 {
            tunnel: w349 -> [_ w354]
            frame False {
            }
            frame True {
              n125 = case shown="True" w354 {
                tunnel: [Bits_to_Write."DBS off" ("Bits to write") Bits_to_Write."DBS on" ("Bits to write")] -> w352
                frame False {
                }
                frame True {
                }
              }
              n126 = local read "DO Task"() -> (w353:refnum<k21>)
              n127 = call "WriteDigioBits2_DAQmx.vi"("Bits to write"=w352, "DO Task"=w353) -> ()  [unwired: 9 in, 1 out]
            }
          }
        }
        n128 = Or(x="Read Settings", y=w333) -> (x .or. y?=w334:bool)
        n129 = Wait Until Next ms Multiple(millisecond multiple=u32 50) -> ()  [unwired: 1 out]
        n130 = case shown="True" w334 {
          tunnel: w333 -> [_ w411]
          frame False {
          }
          frame True {
            n131 = local read "next trial path"() -> (w412:path)
            n132 = case shown="True" w411 {
              tunnel: [enum16{"Query & Read", "Assign & Read", "Write"}."Assign & Read" ("Read/write") enum16{"Query & Read", "Assign & Read", "Write"}."Query & Read" ("Read/write")] -> w414
              frame True {
                n133 = local write "Assign settings"(FALSE ("Assign settings")) -> ()
              }
              frame False {
              }
            }
            n134 = call "ReadWriteSettingsFile4.vi"("file path"=w412, "Read/write"=w414) -> ("Settings Out"=w432:T6, "current path"=→"current path":path)  [unwired: 4 in, 2 out]
            n135 = Unbundle By Name(w432) -> ("Pre-I hold"=w431:cluster{"Fixed (s)":dbl, "Random (s)":dbl}, "LED I duration"=w430:cluster{"Fixed (s)":dbl, "Random (s)":dbl}, "All Flash?"=w429:bool, "Pre-cue brightness"=w428:i16, "Post-I hold"=w427:cluster{"Fixed (s)":dbl, "Random (s)":dbl}, "Post-I \nbounce-off"=w426:cluster{"Fixed (s)":dbl, "Random (s)":dbl}, "Capture timeout"=w425:cluster{"Fixed (s)":dbl, "Random (s)":dbl}, "Tone duration"=w424:cluster{"Fixed (s)":dbl, "Random (s)":dbl}, "LED C duration"=w423:cluster{"Fixed (s)":dbl, "Random (s)":dbl}, "Cue brightness"=w422:i16, "Hold duration"=w421:cluster{"Fixed (s)":dbl, "Random (s)":dbl}, "Allowed\nbounce-off"=w420:cluster{"Fixed (s)":dbl, "Random (s)":dbl}, "Post-capture brightness"=w419:i16, "Reward duration"=w418:cluster{"Fixed (s)":dbl, "Random (s)":dbl}, "Intertrial interval"=w417:cluster{"Fixed (s)":dbl, "Random (s)":dbl}, "Persistent Mode?"=w416:bool, "Error bong?"=w415:bool, "Critter"=w410:u16, "Target set"=w409:i16[], "Rand/Seq?"=w408:bool, "Trial type"=w407:u16, "Sines?"=w406:bool, "Bumps"=w405:bool, "Sine parameters"=w404:T4, "Bump timing"=w403:cluster{"Fix":dbl, "Rnd":dbl}, "Bump Parameters"=w402:T3, "DBS On?"=w401:bool, "Home reward?"=w400:bool, "Home+target OK?"=w399:bool)
            n136 = local write "Pre-I hold"(w431) -> ()
            n137 = local write "All Flash?"(w429) -> ()
            n138 = local write "Post-I hold"(w427) -> ()
            n139 = local write "Capture timeout"(w425) -> ()
            n140 = local write "LED C duration"(w423) -> ()
            n141 = local write "Hold duration"(w421) -> ()
            n142 = local write "Post-capture brightness"(w419) -> ()
            n143 = local write "Intertrial interval"(w417) -> ()
            n144 = local write "Error\nbong?"(w415) -> ()
            n145 = local write "Target set"(w409) -> ()
            n146 = local write "Trial type"(w407) -> ()
            n147 = local write "Home+target OK?"(w399) -> ()
            n148 = local write "DBS On?"(w401) -> ()
            n149 = local write "Bumps"(w405) -> ()
            n150 = local write "Bump delay"(w403) -> ()
            n151 = local write "Sine parameters"(w404) -> ()
            n152 = local write "Bump Parameters"(w402) -> ()
            n153 = local write "Home reward?"(w400) -> ()
            n154 = local write "Rand/Seq?"(w408) -> ()
            n155 = local write "Persistent\n Mode?"(w416) -> ()
            n156 = local write "LED I duration"(w430) -> ()
            n157 = local write "Pre-cue brightness"(w428) -> ()
            n158 = local write "Post-I \nbounce-off"(w426) -> ()
            n159 = local write "Tone duration"(w424) -> ()
            n160 = local write "Cue brightness"(w422) -> ()
            n161 = local write "Allowed\nbounce-off"(w420) -> ()
            n162 = local write "Reward duration"(w418) -> ()
            n163 = local write "Critter"(w410) -> ()
            n164 = local write "Sines?"(w406) -> ()
          }
        }
        n165 = call-poly <vilib>:"Sound Output Set Volume.vi"("error in (no error)"=w305, "volume"="Volume", "task ID"=w306) -> ("error out"=w310:errorcluster, "task ID out"=w309:T11)  [unwired: 7 in]
        n166 = local read "DI Task"() -> (w342:refnum<k21>)
        n167 = local read "Touch lines"() -> (w341:T8)
        n168 = call "CheckAllTouchSensors.vi"("Touch sensor lines"=w341, "DI Task"=w342) -> ("TS 4"=→"TS 4":bool, "TS 3"=→"TS 3":bool, "TS 2"=→"TS 2":bool, "TS 1"=→"TS 1":bool, "Home?"=w302:bool)
        "TS Home" <- w302
        n169 = case shown="False" w302 {
          tunnel: [0.0 ("Frequency") "Frequency"] -> w312
          tunnel: [0.0 ("amplitude") w346] -> w301
          frame False {
          }
          frame True {
            w346 = 1.0  # amplitude
          }
        }
        n170 = call <vilib>:"Sine Waveform.vi"("sampling info"=w307, "amplitude"=w301, "frequency"=w312) -> ("signal out"=w311:waveform(dbl))  [unwired: 7 in, 1 out]
        n171 = call-poly <vilib>:"Sound Output Write.vi"("error in (no error)"=w310, "data"=w311, "task ID"=w309) -> ("error out"=w303:errorcluster, "task ID out"=w304:T11)  [unwired: 7 in]
        n172 = local read "DO Task"() -> (w316:refnum<k21>)
        n173 = call "Control Motor.vi"("Sines?"="Sines?", "Command"=enum16{"Initialize", "Home", "Run", "Disable"}."Run", "Re-center\nmotor"="Recenter motor", "DO Task"=w316, "Sine parameters"="Sine parameters", "Override bumps"="Override bumps", "Home"="Home", "Bumps"="Bumps", "Bump timing"="Bump delay", "Start bump timer?"="Start bump timer?", "Bump Parameters"="Bump Parameters") -> ("Reset\nrecenter"=w318:bool, "Reset override bumps"=w320:bool, "Reset start button"=w322:bool)  [unwired: 2 in]
        n174 = local write "Start bump timer?"(w322) -> ()
        n175 = local write "Recenter motor"(w318) -> ()
        n176 = local write "Override bumps"(w320) -> ()
      }
      n177 = while {
        stop <- w62 stop-if-true
        # "Loop--cycle through all blocks in list until all blocks are completed"
        n178 = stacked-sequence {
          tunnel: [_ _ _ _ w287] -> w65
          tunnel: [_ _ w279 _ _] -> w63
          frame #0 {
            n179 = local read "Exp reset"() -> (w262:bool)
            n180 = case shown="True" w262 {
              frame False {
              }
              frame True {
                n181 = stacked-sequence {
                  frame #0 {
                    n182 = call <vilib>:"Beep.vi"() -> ()  [unwired: 12 in]
                    n183 = Wait (ms)(milliseconds to wait=u32 5) -> ()  [unwired: 1 out]
                  }
                  frame #1 {
                    n184 = local write "Exp reset"(FALSE ("Exp reset")) -> ()
                  }
                  frame #2 {
                    n185 = local write "target set #"(0 ("target set #")) -> ()
                  }
                  frame #3 {
                    n186 = call "TrackStats2.vi"("Command"=T13."Reset for exp") -> ("Total incorrect"=w275:i32, "Total correct"=w274:i32, "# total trials"=w273:i32, "Total % correct"=w272:dbl, "Segment trials"=w271:i32, "Experiment trials"=w268:i32, "Experiment correct"=w266:i32, "Experiment %"=w269:dbl, "Segment Percentage"=w270:dbl)  [unwired: 6 in]
                    n187 = local write "Exp trials"(w268) -> ()
                    n188 = local write "Total incorrect"(w275) -> ()
                    n189 = local write "Total correct"(w274) -> ()
                    n190 = local write "Exp %"(w269) -> ()
                    n191 = local write "Exp correct"(w266) -> ()
                    n192 = local write "Block %"(w270) -> ()
                    n193 = local write "Block trials"(w271) -> ()
                    n194 = local write "Total trials"(w273) -> ()
                    n195 = local write "Total %"(w272) -> ()
                  }
                }
              }
            }
          }
          frame #1 {
            n196 = local read "target set #"() -> (w276:i32)
            n197 = Increment(x=w276) -> (x+1=w277:i32)
            n198 = local write "target set #"(w277) -> ()
          }
          frame #2 {
            n199 = local read "target set #"() -> (w284:i32)
            n200 = call "GetSettingsFileFromTargetSetNum.vi"("target set #"=w284, "# Cycles"="# Cycles", "Block"="Block") -> ("# target sets"=→"# target sets":u16, "Completed list?"=w279:bool, "apply new settings?"=→"Assign settings":bool, "Settings file"=→"next trial path":path)  [unwired: 1 in]
          }
          frame #3 {
            n201 = local read "Assign settings"() -> (w285:bool)
            n202 = case shown="True" w285 {
              frame False {
              }
              frame True {
                # "500ms delay to allow \nsettings loop below to\ninstantiate new settings"
                n203 = Wait (ms)(milliseconds to wait=u32 500) -> ()  [unwired: 1 out]
              }
            }
          }
          frame #4 {
            n204 = call "TargetOverride.vi"("Override 1"="Override 1", "Override 2"="Override 2", "Override 3"="Override 3", "Override 4"="Override 4", "Target set"="Target set") -> ("Target set out"=w293:i16[])  [unwired: 1 in]
            n205 = case shown="True" "Rand/Seq?" {
              tunnel: w293 -> [w297 w299]
              tunnel: [w297 w298] -> w288
              frame False {
              }
              frame True {
                n206 = call "RandomizeTargetSet.vi"("Target set"=w299) -> ("Target set rand order"=w298:i16[])
              }
            }
            n207 = Increment(x=w288) -> (x+1=w287:i16[])
            n208 = Array Size(array=w287) -> (size(s)=→"target set size":i32)
          }
        }
        n209 = local read "stop"() -> (w64:bool)
        n210 = while {
          tunnel: w65 -> [w74] mode=indexing
          tunnel: w65 -> [w73]
          i -> [w72]
          stop <- w66 stop-if-true
          # "Loop--do each target in set until target set is completed"
          n211 = Array Size(array=w73) -> (size(s)=w71:i32)
          n212 = Increment(x=w72) -> (x+1=w70:i32)
          n213 = Greater Or Equal?(x=w70, y=w71) -> (x >= y?=w68:bool)
          n214 = local read "stop"() -> (w69:bool)
          n215 = while {
            shift-right: [w82] -> _
            shift-left: T9."Pre-instruction hold init" ("Current stage") -> [w81]
            tunnel: w74 -> [w80]
            stop <- w77 stop-if-true
            # "Loop--go through each stage of trial until trial is completed"
            n216 = case shown="\"Reward stage\"" w81 {
              tunnel: [T9."Pre-instruction hold" ("Current stage") w91 T9."Instruction" ("Current stage") w139 w147 w159 T9."Target capture" ("Current stage") w179 T9."Target hold" ("Current stage") w197 T9."Intertrial" ("Current stage") T9."Pre-instruction hold init" ("Current stage")] -> w82
              tunnel: [FALSE ("Just initialized\nhold loop?") w89 FALSE ("End of trial") FALSE ("End of trial") FALSE ("End of trial") FALSE ("End of trial") FALSE ("End of trial") FALSE ("End of trial") FALSE ("End of trial") FALSE ("End of trial") FALSE ("End of trial") w246] -> w79
              tunnel: w80 -> [_ _ w106 _ _ _ _ _ _ _ _ _]
              frame "Pre-instruction hold init", Default {
                n217 = call "CalculateFixedPlusRandom2.vi"("Component times"="Pre-I hold") -> ("Composite time"=→"Pre-I hold":dbl)  [unwired: 1 in, 1 out]
                "Touching target\nlast time?" <- FALSE ("Touching target\nlast time?")
                "Just initialized\nhold loop?" <- TRUE ("Just initialized\nhold loop?")
              }
              frame "Pre-instruction hold" {
                n218 = case shown="False" "pause" {
                  tunnel: [w102 T9."Pre-instruction hold init" ("Current stage")] -> w91
                  frame False {
                    n219 = local read "Just initialized\nhold loop?"() -> (w97:bool)
                    n220 = local read "Touching target\nlast time?"() -> (w99:bool)
                    n221 = local read "Touch lines"() -> (w100:T8)
                    n222 = local read "Pre-I hold"() -> (w101:dbl)
                    n223 = local read "DO Task"() -> (w93:refnum<k21>)
                    n224 = local read "DI Task"() -> (w92:refnum<k21>)
                    n225 = call "LookForPreInstHold.vi"("Home reward"="Home  reward", "Home reward?"="Home reward?", "DI Task"=w92, "Touch lines"=w100, "Touching home\nlast time?"=w99, "Just initialized\nhold loop?"=w97, "Composite time"=w101, "DO Task"=w93) -> ("Touching home\nthis time?"=w98:bool, "Just initialized\nhold loop out?"=w96:bool, "Next stage in trial"=w102:T9)  [unwired: 1 in]
                    n226 = local write "Touching target\nlast time?"(w98) -> ()
                    n227 = local write "Just initialized\nhold loop?"(w96) -> ()
                  }
                  frame True {
                    n228 = while {
                      stop <- w104 continue-if-true
                      n229 = local read "pause"() -> (w104:bool)
                      n230 = Wait (ms)(milliseconds to wait=u32 100) -> ()  [unwired: 1 out]
                    }
                  }
                }
                n231 = local read "Exp reset"() -> (w89:bool)
              }
              frame "Instruction init" {
                n232 = stacked-sequence {
                  tunnel: w106 -> [_ _ w116 w117 _ _ _]
                  frame #0 {
                    n233 = local read "DO Task"() -> (w109:refnum<k21>)
                    n234 = call "WriteDigioBits2_DAQmx.vi"("Bits to write"=Bits_to_Write."In trial on", "DO Task"=w109) -> ()  [unwired: 9 in, 1 out]
                  }
                  frame #1 {
                    n235 = local read "Record flag"() -> (w111:bool)
                    n236 = case shown="True" w111 {
                      frame False {
                      }
                      frame True {
                        n237 = local read "Exp trials"() -> (w115:i32)
                        n238 = local read "DO Task"() -> (w113:refnum<k21>)
                        n239 = Increment(x=w115) -> (x+1=w112:i32)
                        n240 = call "WriteDigioBits2_DAQmx.vi"("Bits to write"=Bits_to_Write."Trial number", "Number"=w112, "DO Task"=w113) -> ()  [unwired: 8 in, 1 out]
                      }
                    }
                  }
                  frame #2 {
                    "Target" <- w116
                  }
                  frame #3 {
                    n241 = local read "DO Task"() -> (w118:refnum<k21>)
                    n242 = call "WriteDigioBits2_DAQmx.vi"("Bits to write"=Bits_to_Write."Target number", "Number"=w117, "DO Task"=w118) -> ()  [unwired: 8 in, 1 out]
                  }
                  frame #4 {
                    n243 = case shown="1" "Trial type" {
                      tunnel: [Bits_to_Write."Trial type preQ off" ("Bits to write") Bits_to_Write."Trial type preQ on" ("Bits to write")] -> w120
                      frame 0, Default {
                        # "Trial type = all flash"
                      }
                      frame 1 {
                        # "Trial type = precue"
                      }
                    }
                    n244 = local read "DO Task"() -> (w121:refnum<k21>)
                    n245 = call "WriteDigioBits2_DAQmx.vi"("Bits to write"=w120, "DO Task"=w121) -> ()  [unwired: 9 in, 1 out]
                  }
                  frame #5 {
                    n246 = call "CalculateFixedPlusRandom2.vi"("Component times"="LED I duration") -> ("Composite time"=w125:dbl)  [unwired: 1 in, 1 out]
                    "Instruct duration" <- w125
                    n247 = Greater Than 0?(x=w125) -> (x > 0?=w126:bool)
                    n248 = case shown="True" w126 {
                      frame False {
                      }
                      frame True {
                        w133 = TRUE  # Initialize?
                        n249 = local read "Pre-cue brightness"() -> (w131:i16)
                        n250 = local read "All Flash?"() -> (w130:bool)
                        n251 = local read "DO Task"() -> (w129:refnum<k21>)
                        n252 = local read "DI Task"() -> (w128:refnum<k21>)
                        n253 = local read "Target"() -> (w132:i16)
                        n254 = call "Instruction.vi"("Initialize?"=w133, "DI Task"=w128, "All Flash?"=w130, "brightness"=w131, "Target"=w132, "DO Task"=w129) -> ()  [unwired: 4 in, 2 out]
                      }
                    }
                  }
                  frame #6 {
                    n255 = local read "Bumps"() -> (w134:bool)
                    n256 = local write "Start bump timer?"(w134) -> ()
                  }
                }
              }
              frame "Instruction" {
                w144 = FALSE  # Initialize?
                n257 = local read "Instruct duration"() -> (w140:dbl)
                n258 = local read "Touch lines"() -> (w145:T8)
                n259 = local read "DO Task"() -> (w136:refnum<k21>)
                n260 = local read "DI Task"() -> (w135:refnum<k21>)
                n261 = local read "Target"() -> (w142:i16)
                n262 = call "Instruction.vi"("Initialize?"=w144, "DI Task"=w135, "All Flash?"="All Flash?", "Touch lines"=w145, "Instruction duration"=w140, "brightness"="Pre-cue brightness", "Target"=w142, "DO Task"=w136) -> ("Last trial successful?"=w143:bool, "Go to stage"=w139:T9)  [unwired: 2 in]
                n263 = local write "Last trial successful?"(w143) -> ()
              }
              frame "Post-instruction hold init" {
                w151 = TRUE  # Initialize?
                n264 = local read "DI Task"() -> (w152:refnum<k21>)
                n265 = call "LookForPostInstHold.vi"("Initialize?"=w151, "Post-I \nbounce-off"="Post-I \nbounce-off", "Post-I hold"="Post-I hold", "DI Task"=w152) -> ("Last trial successful?"=w150:bool, "Go to stage"=w147:T9)  [unwired: 6 in]
                n266 = local write "Last trial successful?"(w150) -> ()
              }
              frame "Post-instruction hold" {
                w156 = FALSE  # Initialize?
                # "This is to clear our Catch Boolean during\nthe reward cycle. We put it here so it was\non long enough for us to catch."
                n267 = local read "Touch lines"() -> (w158:T8)
                n268 = local read "DI Task"() -> (w157:refnum<k21>)
                n269 = local write "Catch Trial?"(FALSE) -> ()
                n270 = call "LookForPostInstHold.vi"("Initialize?"=w156, "Touch lines"=w158, "DI Task"=w157) -> ("Last trial successful?"=w155:bool, "Go to stage"=w159:T9)  [unwired: 7 in]
                n271 = local write "Last trial successful?"(w155) -> ()
              }
              frame "Target capture init" {
                w169 = TRUE  # Initialize?
                n272 = local read "DO Task"() -> (w161:refnum<k21>)
                n273 = local read "DI Task"() -> (w160:refnum<k21>)
                n274 = local read "Target"() -> (w167:i16)
                n275 = call "TargetCapture.vi"("DO Task"=w161, "DI Task"=w160, "Response time"="Capture timeout", "Tone duration"="Tone duration", "LED C duration"="LED C duration", "Target"=w167, "Cue brightness"="Cue brightness", "Initialize?"=w169) -> ("Last trial successful?"=w165:bool)  [unwired: 6 in, 1 out]
                n276 = local write "Last trial successful?"(w165) -> ()
              }
              frame "Target capture" {
                w175 = FALSE  # Initialize?
                n277 = local read "Touch lines"() -> (w176:T8)
                n278 = local read "DO Task"() -> (w172:refnum<k21>)
                n279 = local read "DI Task"() -> (w171:refnum<k21>)
                n280 = local read "Target"() -> (w178:i16)
                n281 = call "TargetCapture.vi"("DO Task"=w172, "Touch lines"=w176, "DI Task"=w171, "Home+target OK?"="Home+target OK?", "Target"=w178, "Initialize?"=w175) -> ("Go to stage"=w179:T9, "Last trial successful?"=w177:bool)  [unwired: 8 in]
                n282 = local write "Last trial successful?"(w177) -> ()
              }
              frame "Target hold init" {
                w185 = TRUE  # Initialize?
                n283 = local read "DO Task"() -> (w181:refnum<k21>)
                n284 = local read "DI Task"() -> (w180:refnum<k21>)
                n285 = local read "Target"() -> (w183:i16)
                n286 = call "TargetHold.vi"("DO Task"=w181, "DI Task"=w180, "target hold"="Hold duration", "target\nbounce-off"="Allowed\nbounce-off", "Target"=w183, "Post-capture brightness"="Post-capture brightness", "Initialize?"=w185) -> ()  [unwired: 7 in, 2 out]
              }
              frame "Target hold" {
                w192 = FALSE  # Initialize?
                n287 = local read "Home+target OK?"() -> (w190:bool)
                n288 = local read "Touch lines"() -> (w195:T8)
                n289 = local read "DO Task"() -> (w196:refnum<k21>)
                n290 = local read "DI Task"() -> (w189:refnum<k21>)
                n291 = local read "Target"() -> (w194:i16)
                n292 = call "TargetHold.vi"("DO Task"=w196, "Touch lines"=w195, "DI Task"=w189, "Home+target OK?"=w190, "Target"=w194, "Initialize?"=w192) -> ("Go to stage"=w197:T9, "Last trial successful?"=w193:bool)  [unwired: 8 in]
                n293 = local write "Last trial successful?"(w193) -> ()
              }
              frame "Reward stage" {
                n294 = flat-sequence {
                  frame #0 {
                    # "This is the Catch Trial bit to write\nto file."
                    # "This will be a bit written in the \ndata file so we're not worried about \nit reseting."
                    n295 = Random Number (0-1)() -> (number: 0 to 1=w211:dbl)
                    n296 = Multiply(x=w211, y=100.0) -> (x*y=w210:dbl)
                    n297 = To Unsigned Long Integer(number=w210) -> (unsigned 32bit integer=w209:u32)
                    n298 = Less Or Equal?(x=w209, y="Catch probability") -> (x <= y?=w208:bool)
                    n299 = Not Equal To 0?(x="Catch probability") -> (x != 0?=w207:bool)
                    n300 = And(x=w208, y=w207) -> (x .and. y?=w205:bool)
                    n301 = case shown="True" w205 {
                      selector: w205 -> [w216 w218]
                      tunnel: ["Reward duration" cluster{"Fix":dbl, "Rnd":dbl} {"Fix"=0.0, "Rnd"=0.0} ("Reward duration")] -> w214
                      tunnel: [w216 w218] -> w200
                      frame False {
                        # "Sending False bit for \ncatch trial"
                        # "Normal reward duration"
                      }
                      frame True {
                        # "Sending True bit for \ncatch trial"
                        # "This is the catch trial. \nSo we don't want to deliver \na reward"
                      }
                    }
                    "Catch Trial?" <- w200
                    n302 = call "CalculateFixedPlusRandom2.vi"("Component times"=w214) -> ("time in ms"=w215:dbl)  [unwired: 1 in, 1 out]
                    n303 = local read "DO Task"() -> (w213:refnum<k21>)
                    n304 = call "Reward Pulse.vi"("Pulse duration (ms)"=w215, "DO Task"=w213) -> ()  [unwired: 8 in]
                    n305 = Select(t=Bits_to_Write."LED 4 on" ("Bits to write"), s=w200, f=Bits_to_Write."LED 4 off" ("Bits to write")) -> (s? t:f=w201:T12)
                    n306 = call "WriteDigioBits2_DAQmx.vi"("Bits to write"=w201, "DO Task"=refnum<k21> "BlueSimple_DO_All" ("DO Task 2")) -> ()  [unwired: 9 in, 1 out]
                  }
                  frame #1 {
                    # "This second sequence is for the Arm Freeze Reward Timer.\nWhen the monkey reaches to the target, her arm freezes.\nThis routine provides a timer to notify the tirainer to give \nthe monkey a treat and return her arm to the home key."
                    n307 = case shown="True" "Arm Freeze \nCounter" {
                      frame False {
                      }
                      frame True {
                        n308 = flat-sequence {
                          frame #0 {
                            n309 = Multiply(x="Time to wait\nbefore treat \nArm freeze (S)", y=1000) -> (x*y=w221:dbl)
                            n310 = Wait (ms)(milliseconds to wait=w221) -> ()  [unwired: 1 out]
                          }
                          frame #1 {
                            n311 = call <vilib>:"Beep.vi"("use system alert? (T)"=TRUE) -> ()  [unwired: 11 in]
                          }
                        }
                      }
                    }
                  }
                }
              }
              frame "Intertrial" {
                n312 = local read "Last trial successful?"() -> (w242:bool)
                n313 = local read "Bumps"() -> (w226:bool)
                n314 = local read "target set size"() -> (w230:i32)
                n315 = local read "# target sets"() -> (w231:u16)
                n316 = call "CalculateFixedPlusRandom2.vi"("Component times"="Intertrial interval") -> ("Composite time"=w243:dbl)  [unwired: 1 in, 1 out]
                n317 = local write "Override bumps"(w226) -> ()
                n318 = local write "Recenter motor"(w226) -> ()
                n319 = while {
                  shift-right: [enum16{"Start counting", "Read count", "Reset"}."Read count" ("Enum")] -> _
                  shift-left: enum16{"Start counting", "Read count", "Reset"}."Start counting" ("Enum") -> [w261]
                  tunnel: [w256] -> _
                  tunnel: w243 -> [w255]
                  stop <- w257 stop-if-true
                  n320 = call "non-Reentrant Controllable Timer.vi"("Enum"=w261) -> ("Time out"=w259:dbl)  [unwired: 1 in]
                  n321 = local read "stop"() -> (w258:bool)
                  n322 = Greater Or Equal?(x=w259, y=w255) -> (x >= y?=w256:bool)
                  n323 = Or(x=w256, y=w258) -> (x .or. y?=w257:bool)
                }
                n324 = Multiply(x=w231, y=w230) -> (x*y=w229:i32)
                n325 = call "TrackStats2.vi"("Last trial successful?"=w242, "Trial bin size"=w229, "Persistent\n Mode?"="Persistent\n Mode?", "Command"=enum16{"Reset", "Increment"}."Increment") -> ("Total incorrect"=→"Total incorrect":i32, "Total correct"=→"Total correct":i32, "# total trials"=→"Total trials":i32, "Total % correct"=w234:dbl, "Segment trials"=→"Block trials":i32, "Experiment trials"=→"Exp trials":i32, "Experiment correct"=→"Exp correct":i32, "Experiment %"=→"Exp %":dbl, "Segment Percentage"=w235:dbl)  [unwired: 3 in]
                "Block %" <- w235
                "Total %" <- w234
                n326 = Bundle("Segment Percentage"=w235, "Total % correct"=w234) -> (→"Waveform Chart":T7)  [unwired: 1 in]
                n327 = stacked-sequence {
                  frame #0 {
                    n328 = local read "Last trial successful?"() -> (w248:bool)
                    n329 = case shown="True" w248 {
                      frame False {
                        n330 = local read "DO Task"() -> (w249:refnum<k21>)
                        n331 = call "Signal Error.vi"("DO Task"=w249, "Error bong?"="Error\nbong?") -> ()  [unwired: 3 in]
                      }
                      frame True {
                      }
                    }
                  }
                  frame #1 {
                    n332 = local read "DO Task"() -> (w251:refnum<k21>)
                    n333 = call "WriteDigioBits2_DAQmx.vi"("Bits to write"=Bits_to_Write."In trial off", "DO Task"=w251) -> ()  [unwired: 9 in, 1 out]
                  }
                  frame #2 {
                  }
                }
                n334 = local read "Persistent\n Mode?"() -> (w232:bool)
                n335 = case shown="False" w232 {
                  tunnel: [w253 w254] -> w246
                  frame False {
                    w253 = TRUE  # End of trial
                  }
                  frame True {
                    n336 = local read "Last trial successful?"() -> (w254:bool)
                  }
                }
              }
            }
            n337 = Wait (ms)(milliseconds to wait=u32 1) -> ()  [unwired: 1 out]
            n338 = Compound Arithmetic op=OR(w79, "stop") -> (w77:bool)
            "Current stage" <- w81
          }
          n339 = local read "Exp reset"() -> (w67:bool)
          n340 = Compound Arithmetic op=OR(w69, w68, w67) -> (w66:bool)
        }
        n341 = Or(x=w64, y=w63) -> (x .or. y?=w62:bool)
      }
      n342 = call <vilib>:"Sound Output Clear.vi"("error in (no error)"=w56, "task ID"=w57) -> ("error out"=w58:errorcluster)  [unwired: 9 in]
      n343 = call <vilib>:"Simple Error Handler.vi"("error in (no error)"=w58) -> ()  [unwired: 4 in, 5 out]
    }
    frame #3 {
      # "Turn LED's, \nbuzzer,\npump off\njust to be\nsure"
      n344 = local read "DO Task"() -> (w449:refnum<k21>)
      n345 = local read "DO Task"() -> (w447:refnum<k21>)
      n346 = local read "DO Task"() -> (w451:refnum<k21>)
      n347 = local read "DO Task"() -> (w452:refnum<k21>)
      n348 = local read "DO Task"() -> (w454:refnum<k21>)
      n349 = local read "DO Task"() -> (w456:refnum<k21>)
      n350 = local write "Record flag"(FALSE ("Record flag")) -> ()
      n351 = call "WriteDigioBits2_DAQmx.vi"("Bits to write"=Bits_to_Write."In trial off", "DO Task"=w449) -> ()  [unwired: 9 in, 1 out]
      n352 = call "WriteDigioBits2_DAQmx.vi"("Bits to write"=Bits_to_Write."All LEDs off", "DO Task"=w447) -> ()  [unwired: 9 in, 1 out]
      n353 = call "WriteDigioBits2_DAQmx.vi"("Bits to write"=Bits_to_Write."Buzzer off", "DO Task"=w451) -> ()  [unwired: 9 in, 1 out]
      n354 = call "WriteDigioBits2_DAQmx.vi"("Bits to write"=Bits_to_Write."Reward off", "DO Task"=w452) -> ()  [unwired: 9 in, 1 out]
      n355 = call "WriteDigioBits2_DAQmx.vi"("Bits to write"=Bits_to_Write."Error off", "DO Task"=w454) -> ()  [unwired: 9 in, 1 out]
      n356 = call "WriteDigioBits2_DAQmx.vi"("Bits to write"=Bits_to_Write."DBS off", "DO Task"=w456) -> ()  [unwired: 9 in, 1 out]
      n357 = local write "stop"(FALSE ("stop")) -> ()
    }
  }
